vi "Hexapod_pressure_GUI.vi"() -> ()   [LabVIEW 2011]
panel:
  out "pressure read 9":dbl
  in  "pressure read 8":dbl
  out "pressure read 7":dbl
  in  "pressure read 4":dbl
  in  "M4StageNeg":bool
  in  "M4StagePos":bool
  in  "OAP1StageNeg":bool
  in  "OAP1StagePos":bool
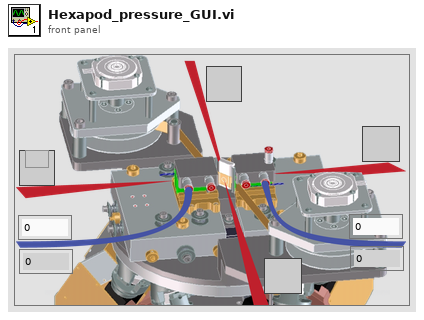
[diagram p1: front panel]
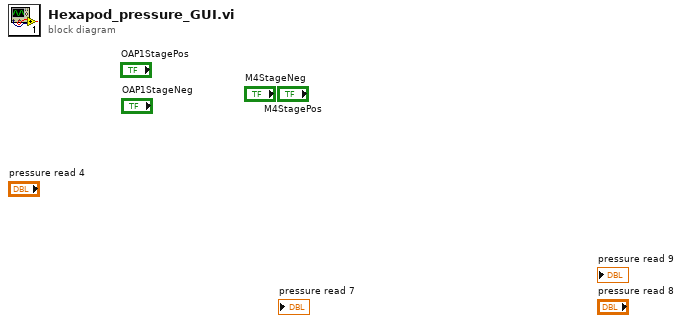
[diagram p0: block diagram]
diagram:
